vi "binaryzation.vi"() -> ()   [LabVIEW 2014]
panel:
  out "image out":T1(plugin-control)
  out "Src":T1(plugin-control)
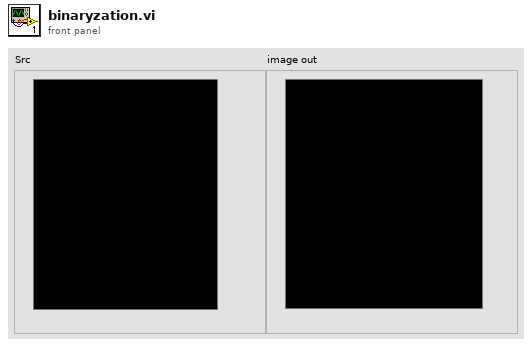
[diagram p1: front panel]
types:
  T1 = typedef "IMAQ Image.ctl" = refnum<image>
  T2 = typedef "Image Type" = u32
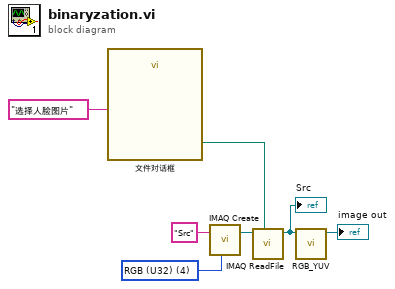
[diagram p0: block diagram]
diagram:
  w7 = T2 4 items=["Grayscale (U8)", "Grayscale (I16)", "Grayscale (SGL)", "Complex (CSG)", "RGB (U32)", "HSL (U32)", "RGB (U64)", "Grayscale (U16)"] ("Src")
  n1 = call "文件对话框"("prompt"="选择人脸图片") -> ("selected path"=w1:path)  [unwired: 11 in, 3 out]
  n2 = call "IMAQ Create"("Image Name"="Src", "Image Type"=w7) -> ("New Image"=w5:T1)  [unwired: 3 in, 1 out]
  n3 = call "IMAQ ReadFile"("File Path"=w1, "Image"=w5) -> ("Image Out"=w4:T1)  [unwired: 5 in, 4 out]
  "Src" <- w4
  n4 = call "RGB_YUV.vi"("Image In"=w4) -> ("Image Out"=→"image out":T1)  [unwired: 9 in, 1 out]
